vi "Coerce Value.vi"(8 "error in (no error)":errorcluster, 9 "Value":variant, 10 "ParamTags":T1, 11 "Waveforms Common Methods in":refnum<class "Waveforms Common Methods.lvclass">) -> (0 "error out":errorcluster, 1 "Coerced Value":variant, 3 "Waveforms Common Methods out":refnum<class "Waveforms Common Methods.lvclass">)   [LabVIEW 2021, in "Rigol DG822 UI.lvlib" / "Waveforms Common Methods.lvclass"]
uses:
  Waveforms Common Methods.lvclass
  lib/controls.llb/WaveformParamTags.ctl
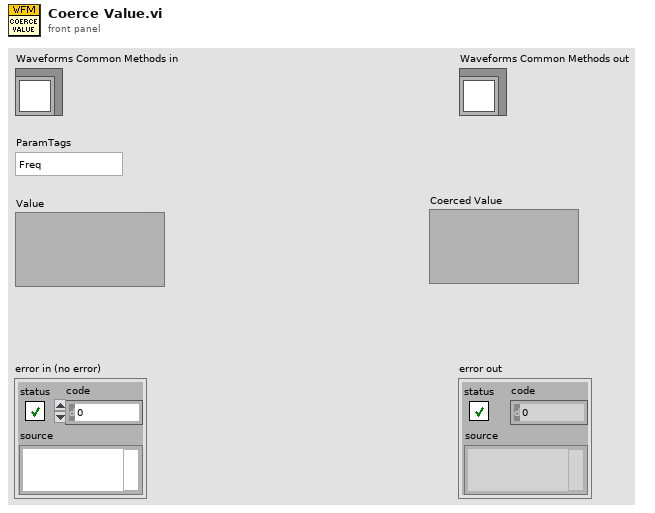
[diagram p1: front panel]
types:
  T1 = typedef "WaveformParamTags.ctl" = enum16{"Freq", "Period", "Ampl", "HighL", "Offset", "LowL", "Phase", "Duty", "Width", "RisEdge", "FallEdge"}
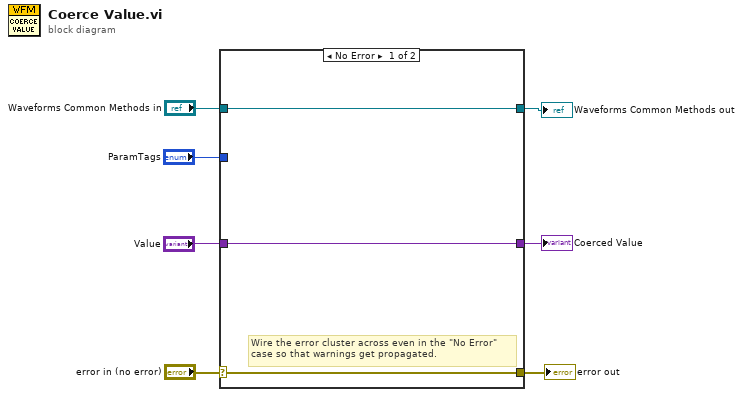
[diagram p0: block diagram]
diagram:
  n1 = case shown="No Error" "error in (no error)" {
    selector: "error in (no error)" -> [w9 w12]
    tunnel: [w9 w12] -> w6
    tunnel: [w10 w11] -> w4
    tunnel: "Waveforms Common Methods in" -> [w10 w11]
    tunnel: "ParamTags" -> [_ _]
    tunnel: [w8 _] -> w2
    tunnel: "Value" -> [w8 _]
    frame No Error {
      # "Wire the error cluster across even in the \"No Error\"\ncase so that warnings get propagated."
    }
    frame Error {
    }
  }
  "error out" <- w6
  "Waveforms Common Methods out" <- w4
  "Coerced Value" <- w2
